vi "toml_api_resolve_path.vi"(1 "path":path) -> (0 "resolved path":path)   [LabVIEW 2017]
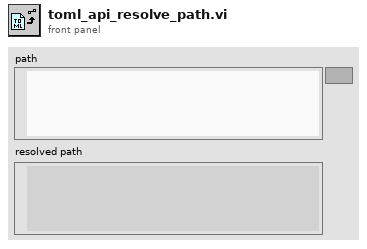
[diagram p1: front panel]
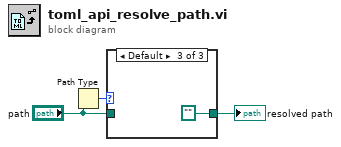
[diagram p0: block diagram]
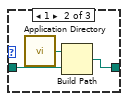
[diagram p3: hidden frame]
diagram:
  n1 = Path Type(1:"path") -> (0:w1:i16)
  n2 = case shown="Default" w1 {
    tunnel: "path" -> [w4 w6 _]
    tunnel: [w4 w5 path ""] -> w2
    frame 0 {
    }
    frame 1 {
      n3 = call <vilib>:"Application Directory.vi"() -> ("Application Directory"=w7:path)
      n4 = Build Path(base path=w7, name or relative path=w6) -> (appended path=w5:path)
    }
    frame Default {
    }
  }
  "resolved path" <- w2
